vi "S4GUI_001.vi"() -> ()   [LabVIEW 2018] (continued)
  T9 = cluster{"Trigger Mode Status":string, "String output":string, "Instrument Status":cluster{"WPROT pos":dbl, "WPSEL pos":dbl, "GMIR pos":dbl, "GFOC pos":dbl, "CALW pos":dbl, "ASEL pos":dbl, "connection":bool, "mode":bool, "String Status":string}, "Sync Box State":i32, "Trigger General Status":string, "Instrument States":cluster{"WPSEL State":i32, "WPROT State":i32, "CALW State":i32, "ASEL State":i32, "GMIR State":i32, "GFOC State":i32}, "Instrument Pos Names":cluster{"WPROT posname":string, "WPSEL posname":string, "CALW posname":string, "ASEL posname":string}, "ChannelA_Status":cluster{"Current exp":dbl, "Frames done":u32, "LastFileImage":string, "CamStatus":string, "Run state":u32, "connection":bool, "Cooler ON/OFF":i16, "Currently temperature":i16, "Temperature Status":string, "target  temp":i16, "conf runing":bool, "FT":bool}, "WPROT seq":u16, "ChannelB_Status":cluster{"Current exp":dbl, "Frames done":u32, "LastFileImage":string, "CamStatus":string, "Run state":u32, "connection":bool, "Cooler ON/OFF":i16, "Currently temperature":i16, "Temperature Status":string, "target  temp":i16, "conf runing":bool, "FT":bool}, "ChannelC_Status":cluster{"Current exp":dbl, "Frames done":u32, "LastFileImage":string, "CamStatus":string, "Run state":u32, "connection":bool, "Cooler ON/OFF":i16, "Currently temperature":i16, "Temperature Status":string, "target  temp":i16, "conf runing":bool, "FT":bool}, "ChannelD_Status":cluster{"Current exp":dbl, "Frames done":u32, "LastFileImage":string, "CamStatus":string, "Run state":u32, "connection":bool, "Cooler ON/OFF":i16, "Currently temperature":i16, "Temperature Status":string, "target  temp":i16, "conf runing":bool, "FT":bool}, "ChannelA_CCD":cluster{"ACQUISITION_MODE":u8, "TRIGGER_MODE":u8, "READ_MODE":u8, "PREAMP":u8, "READOUT_RATE":u8, "VERTICAL_SHIFT_SPEED":u8, "EM_MODE":u8, "EM_GAIN":u16, "SHUTTER_MODE":u8, "SHUTTER_TTL":u8, "SHUTTER_OPENNING_TIME":u16, "SHUTTER_CLOSING_TIME":u16, "VBIN":u16, "HBIN":u16, "INITIAL_LINE":u16, "INITIAL_COLUMN":u16, "FINAL_LINE":u16, "FINAL_COLUMN":u16, "FRAME_TRANSFER":bool, "VERTICAL_CLOCK_VOLTAGE":u8, "AD_CHANNEL":u32}, "ChannelB_CCD ":cluster{"ACQUISITION_MODE":u8, "TRIGGER_MODE":u8, "READ_MODE":u8, "PREAMP":u8, "READOUT_RATE":u8, "VERTICAL_SHIFT_SPEED":u8, "EM_MODE":u8, "EM_GAIN":u16, "SHUTTER_MODE":u8, "SHUTTER_TTL":u8, "SHUTTER_OPENNING_TIME":u16, "SHUTTER_CLOSING_TIME":u16, "VBIN":u16, "HBIN":u16, "INITIAL_LINE":u16, "INITIAL_COLUMN":u16, "FINAL_LINE":u16, "FINAL_COLUMN":u16, "FRAME_TRANSFER":bool, "VERTICAL_CLOCK_VOLTAGE":u8, "AD_CHANNEL":u32}, "ChannelC_CCD":cluster{"ACQUISITION_MODE":u8, "TRIGGER_MODE":u8, "READ_MODE":u8, "PREAMP":u8, "READOUT_RATE":u8, "VERTICAL_SHIFT_SPEED":u8, "EM_MODE":u8, "EM_GAIN":u16, "SHUTTER_MODE":u8, "SHUTTER_TTL":u8, "SHUTTER_OPENNING_TIME":u16, "SHUTTER_CLOSING_TIME":u16, "VBIN":u16, "HBIN":u16, "INITIAL_LINE":u16, "INITIAL_COLUMN":u16, "FINAL_LINE":u16, "FINAL_COLUMN":u16, "FRAME_TRANSFER":bool, "VERTICAL_CLOCK_VOLTAGE":u8, "AD_CHANNEL":u32}, "ChannelD_CCD":cluster{"ACQUISITION_MODE":u8, "TRIGGER_MODE":u8, "READ_MODE":u8, "PREAMP":u8, "READOUT_RATE":u8, "VERTICAL_SHIFT_SPEED":u8, "EM_MODE":u8, "EM_GAIN":u16, "SHUTTER_MODE":u8, "SHUTTER_TTL":u8, "SHUTTER_OPENNING_TIME":u16, "SHUTTER_CLOSING_TIME":u16, "VBIN":u16, "HBIN":u16, "INITIAL_LINE":u16, "INITIAL_COLUMN":u16, "FINAL_LINE":u16, "FINAL_COLUMN":u16, "FRAME_TRANSFER":bool, "VERTICAL_CLOCK_VOLTAGE":u8, "AD_CHANNEL":u32}, "CHA_Checked Params":cluster{"ACQUISITION_MODE":bool, "TRIGGER_MODE":bool, "READ_MODE":bool, "PREAMP":bool, "READOUT_RATE":bool, "VERTICAL_SHIFT_SPEED":bool, "EM_MODE":bool, "EM_GAIN":bool, "SHUTTER_MODE":bool, "SHUTTER_TTL":bool, "SHUTTER_OPENING_TIME":bool, "SHUTTER_CLOSING_TIME":bool, "VBIN":bool, "HBIN":bool, "INITIAL_LINE":bool, "INITIAL_COLUMN":bool, "FINAL_LINE":bool, "FINAL_COLUMN":bool, "FRAME_TRANSFER":bool, "VERTICAL_CLOCK_VOLTAGE":bool, "AD_CHANNEL":bool}, "CHB_Checked Params":cluster{"ACQUISITION_MODE":bool, "TRIGGER_MODE":bool, "READ_MODE":bool, "PREAMP":bool, "READOUT_RATE":bool, "VERTICAL_SHIFT_SPEED":bool, "EM_MODE":bool, "EM_GAIN":bool, "SHUTTER_MODE":bool, "SHUTTER_TTL":bool, "SHUTTER_OPENING_TIME":bool, "SHUTTER_CLOSING_TIME":bool, "VBIN":bool, "HBIN":bool, "INITIAL_LINE":bool, "INITIAL_COLUMN":bool, "FINAL_LINE":bool, "FINAL_COLUMN":bool, "FRAME_TRANSFER":bool, "VERTICAL_CLOCK_VOLTAGE":bool, "AD_CHANNEL":bool}, "CHC_Checked Params":cluster{"ACQUISITION_MODE":bool, "TRIGGER_MODE":bool, "READ_MODE":bool, "PREAMP":bool, "READOUT_RATE":bool, "VERTICAL_SHIFT_SPEED":bool, "EM_MODE":bool, "EM_GAIN":bool, "SHUTTER_MODE":bool, "SHUTTER_TTL":bool, "SHUTTER_OPENING_TIME":bool, "SHUTTER_CLOSING_TIME":bool, "VBIN":bool, "HBIN":bool, "INITIAL_LINE":bool, "INITIAL_COLUMN":bool, "FINAL_LINE":bool, "FINAL_COLUMN":bool, "FRAME_TRANSFER":bool, "VERTICAL_CLOCK_VOLTAGE":bool, "AD_CHANNEL":bool}, "CHD_Checked Params":cluster{"ACQUISITION_MODE":bool, "TRIGGER_MODE":bool, "READ_MODE":bool, "PREAMP":bool, "READOUT_RATE":bool, "VERTICAL_SHIFT_SPEED":bool, "EM_MODE":bool, "EM_GAIN":bool, "SHUTTER_MODE":bool, "SHUTTER_TTL":bool, "SHUTTER_OPENING_TIME":bool, "SHUTTER_CLOSING_TIME":bool, "VBIN":bool, "HBIN":bool, "INITIAL_LINE":bool, "INITIAL_COLUMN":bool, "FINAL_LINE":bool, "FINAL_COLUMN":bool, "FRAME_TRANSFER":bool, "VERTICAL_CLOCK_VOLTAGE":bool, "AD_CHANNEL":bool}, "Trigger_connection":bool, "TCSPD_connection":bool, "TCS extended":string, "TCS id":u32}
  T10 = cluster{"Cluster Mode Sync":cluster{"#Index Cycles":enum8{"Enabled", "Disabled", "Disabled and Grayed Out"}, "#Cycles":enum8{"Enabled", "Disabled", "Disabled and Grayed Out"}, "SSM":enum8{"Enabled", "Disabled", "Disabled and Grayed Out"}, "Set SM":enum8{"Enabled", "Disabled", "Disabled and Grayed Out"}, "Star SM":enum8{"Enabled", "Disabled", "Disabled and Grayed Out"}, "Pause SM":enum8{"Enabled", "Disabled", "Disabled and Grayed Out"}, "Stop SM":enum8{"Enabled", "Disabled", "Disabled and Grayed Out"}, "Abort SM":enum8{"Enabled", "Disabled", "Disabled and Grayed Out"}, "Start SM Text":string}, "Cluster Polarimetry":cluster{"Lambda Selector":enum8{"Enabled", "Disabled", "Disabled and Grayed Out"}, "Calibrator Selector":enum8{"Enabled", "Disabled", "Disabled and Grayed Out"}, "Set Waveplate":enum8{"Enabled", "Disabled", "Disabled and Grayed Out"}, "Select Positions":enum8{"Enabled", "Disabled", "Disabled and Grayed Out"}, "P0":enum8{"Enabled", "Disabled", "Disabled and Grayed Out"}, "P1":enum8{"Enabled", "Disabled", "Disabled and Grayed Out"}, "P2":enum8{"Enabled", "Disabled", "Disabled and Grayed Out"}, "P3":enum8{"Enabled", "Disabled", "Disabled and Grayed Out"}, "P4":enum8{"Enabled", "Disabled", "Disabled and Grayed Out"}, "P5":enum8{"Enabled", "Disabled", "Disabled and Grayed Out"}, "P6":enum8{"Enabled", "Disabled", "Disabled and Grayed Out"}, "P7":enum8{"Enabled", "Disabled", "Disabled and Grayed Out"}, "P8":enum8{"Enabled", "Disabled", "Disabled and Grayed Out"}, "P9":enum8{"Enabled", "Disabled", "Disabled and Grayed Out"}, "P10":enum8{"Enabled", "Disabled", "Disabled and Grayed Out"}, "P11":enum8{"Enabled", "Disabled", "Disabled and Grayed Out"}, "P12":enum8{"Enabled", "Disabled", "Disabled and Grayed Out"}, "P13":enum8{"Enabled", "Disabled", "Disabled and Grayed Out"}, "P14":enum8{"Enabled", "Disabled", "Disabled and Grayed Out"}, "P15":enum8{"Enabled", "Disabled", "Disabled and Grayed Out"}}, "Cluster Mode CH1":cluster{"#cycles ch1":enum8{"Enabled", "Disabled", "Disabled and Grayed Out"}, "Start ch1":enum8{"Enabled", "Disabled", "Disabled and Grayed Out"}, "Pause ch1":enum8{"Enabled", "Disabled", "Disabled and Grayed Out"}, "Stop ch1":enum8{"Enabled", "Disabled", "Disabled and Grayed Out"}, "Abort ch1":enum8{"Enabled", "Disabled", "Disabled and Grayed Out"}, "Exptime ch1":enum8{"Enabled", "Disabled", "Disabled and Grayed Out"}, "Exp ch1":enum8{"Enabled", "Disabled", "Disabled and Grayed Out"}, "Start ch1 Text":string, "Set Cooler":enum8{"Enabled", "Disabled", "Disabled and Grayed Out"}, "Set Temp":enum8{"Enabled", "Disabled", "Disabled and Grayed Out"}}, "Cluster Mode CH2":cluster{"#cycles ch2":enum8{"Enabled", "Disabled", "Disabled and Grayed Out"}, "Start ch2":enum8{"Enabled", "Disabled", "Disabled and Grayed Out"}, "Pause ch2":enum8{"Enabled", "Disabled", "Disabled and Grayed Out"}, "Stop ch2":enum8{"Enabled", "Disabled", "Disabled and Grayed Out"}, "Abort ch2":enum8{"Enabled", "Disabled", "Disabled and Grayed Out"}, "Exptime ch2":enum8{"Enabled", "Disabled", "Disabled and Grayed Out"}, "Exp ch2":enum8{"Enabled", "Disabled", "Disabled and Grayed Out"}, "Start ch2 Text":string, "Set Cooler":enum8{"Enabled", "Disabled", "Disabled and Grayed Out"}, "Set Temp":enum8{"Enabled", "Disabled", "Disabled and Grayed Out"}}, "Cluster Mode CH3":cluster{"#cycles ch3":enum8{"Enabled", "Disabled", "Disabled and Grayed Out"}, "Start ch3":enum8{"Enabled", "Disabled", "Disabled and Grayed Out"}, "Pause ch3":enum8{"Enabled", "Disabled", "Disabled and Grayed Out"}, "Stop ch3":enum8{"Enabled", "Disabled", "Disabled and Grayed Out"}, "Abort ch3":enum8{"Enabled", "Disabled", "Disabled and Grayed Out"}, "Exptime ch3":enum8{"Enabled", "Disabled", "Disabled and Grayed Out"}, "Exp ch3":enum8{"Enabled", "Disabled", "Disabled and Grayed Out"}, "Start ch3 Text":string, "Set Cooler":enum8{"Enabled", "Disabled", "Disabled and Grayed Out"}, "Set Temp":enum8{"Enabled", "Disabled", "Disabled and Grayed Out"}}, "Cluster Mode CH4":cluster{"#cycles ch4":enum8{"Enabled", "Disabled", "Disabled and Grayed Out"}, "Start ch4":enum8{"Enabled", "Disabled", "Disabled and Grayed Out"}, "Pause ch4":enum8{"Enabled", "Disabled", "Disabled and Grayed Out"}, "Stop ch4":enum8{"Enabled", "Disabled", "Disabled and Grayed Out"}, "Abort ch4":enum8{"Enabled", "Disabled", "Disabled and Grayed Out"}, "Exptime ch4":enum8{"Enabled", "Disabled", "Disabled and Grayed Out"}, "Exp ch4":enum8{"Enabled", "Disabled", "Disabled and Grayed Out"}, "Start ch4 Text":string, "Set Cooler":enum8{"Enabled", "Disabled", "Disabled and Grayed Out"}, "Set Temp":enum8{"Enabled", "Disabled", "Disabled and Grayed Out"}}, "Cluster ExpMode":cluster{"tab4":enum8{"Enabled", "Disabled", "Disabled and Grayed Out"}}}
  T11 = cluster{"WPROT pos":dbl, "WPSEL pos":dbl, "GMIR pos":dbl, "GFOC pos":dbl, "CALW pos":dbl, "ASEL pos":dbl, "connection":bool, "mode":bool, "String Status":string}
  T12 = cluster{"WPSEL State":i32, "WPROT State":i32, "CALW State":i32, "ASEL State":i32, "GMIR State":i32, "GFOC State":i32}
  T13 = cluster{"WPROT posname":string, "WPSEL posname":string, "CALW posname":string, "ASEL posname":string}
  T14 = cluster{"Current exp":dbl, "Frames done":u32, "LastFileImage":string, "CamStatus":string, "Run state":u32, "connection":bool, "Cooler ON/OFF":i16, "Currently temperature":i16, "Temperature Status":string, "target  temp":i16, "conf runing":bool, "FT":bool}
  T15 = cluster{"Lambda Selector":enum8{"Enabled", "Disabled", "Disabled and Grayed Out"}, "Calibrator Selector":enum8{"Enabled", "Disabled", "Disabled and Grayed Out"}, "Set Waveplate":enum8{"Enabled", "Disabled", "Disabled and Grayed Out"}, "Select Positions":enum8{"Enabled", "Disabled", "Disabled and Grayed Out"}, "P0":enum8{"Enabled", "Disabled", "Disabled and Grayed Out"}, "P1":enum8{"Enabled", "Disabled", "Disabled and Grayed Out"}, "P2":enum8{"Enabled", "Disabled", "Disabled and Grayed Out"}, "P3":enum8{"Enabled", "Disabled", "Disabled and Grayed Out"}, "P4":enum8{"Enabled", "Disabled", "Disabled and Grayed Out"}, "P5":enum8{"Enabled", "Disabled", "Disabled and Grayed Out"}, "P6":enum8{"Enabled", "Disabled", "Disabled and Grayed Out"}, "P7":enum8{"Enabled", "Disabled", "Disabled and Grayed Out"}, "P8":enum8{"Enabled", "Disabled", "Disabled and Grayed Out"}, "P9":enum8{"Enabled", "Disabled", "Disabled and Grayed Out"}, "P10":enum8{"Enabled", "Disabled", "Disabled and Grayed Out"}, "P11":enum8{"Enabled", "Disabled", "Disabled and Grayed Out"}, "P12":enum8{"Enabled", "Disabled", "Disabled and Grayed Out"}, "P13":enum8{"Enabled", "Disabled", "Disabled and Grayed Out"}, "P14":enum8{"Enabled", "Disabled", "Disabled and Grayed Out"}, "P15":enum8{"Enabled", "Disabled", "Disabled and Grayed Out"}}
  T16 = cluster{"#Index Cycles":enum8{"Enabled", "Disabled", "Disabled and Grayed Out"}, "#Cycles":enum8{"Enabled", "Disabled", "Disabled and Grayed Out"}, "SSM":enum8{"Enabled", "Disabled", "Disabled and Grayed Out"}, "Set SM":enum8{"Enabled", "Disabled", "Disabled and Grayed Out"}, "Star SM":enum8{"Enabled", "Disabled", "Disabled and Grayed Out"}, "Pause SM":enum8{"Enabled", "Disabled", "Disabled and Grayed Out"}, "Stop SM":enum8{"Enabled", "Disabled", "Disabled and Grayed Out"}, "Abort SM":enum8{"Enabled", "Disabled", "Disabled and Grayed Out"}, "Start SM Text":string}
  T17 = cluster{"#cycles ch1":enum8{"Enabled", "Disabled", "Disabled and Grayed Out"}, "Start ch1":enum8{"Enabled", "Disabled", "Disabled and Grayed Out"}, "Pause ch1":enum8{"Enabled", "Disabled", "Disabled and Grayed Out"}, "Stop ch1":enum8{"Enabled", "Disabled", "Disabled and Grayed Out"}, "Abort ch1":enum8{"Enabled", "Disabled", "Disabled and Grayed Out"}, "Exptime ch1":enum8{"Enabled", "Disabled", "Disabled and Grayed Out"}, "Exp ch1":enum8{"Enabled", "Disabled", "Disabled and Grayed Out"}, "Start ch1 Text":string, "Set Cooler":enum8{"Enabled", "Disabled", "Disabled and Grayed Out"}, "Set Temp":enum8{"Enabled", "Disabled", "Disabled and Grayed Out"}}
  T18 = cluster{"#cycles ch2":enum8{"Enabled", "Disabled", "Disabled and Grayed Out"}, "Start ch2":enum8{"Enabled", "Disabled", "Disabled and Grayed Out"}, "Pause ch2":enum8{"Enabled", "Disabled", "Disabled and Grayed Out"}, "Stop ch2":enum8{"Enabled", "Disabled", "Disabled and Grayed Out"}, "Abort ch2":enum8{"Enabled", "Disabled", "Disabled and Grayed Out"}, "Exptime ch2":enum8{"Enabled", "Disabled", "Disabled and Grayed Out"}, "Exp ch2":enum8{"Enabled", "Disabled", "Disabled and Grayed Out"}, "Start ch2 Text":string, "Set Cooler":enum8{"Enabled", "Disabled", "Disabled and Grayed Out"}, "Set Temp":enum8{"Enabled", "Disabled", "Disabled and Grayed Out"}}
  T19 = cluster{"#cycles ch3":enum8{"Enabled", "Disabled", "Disabled and Grayed Out"}, "Start ch3":enum8{"Enabled", "Disabled", "Disabled and Grayed Out"}, "Pause ch3":enum8{"Enabled", "Disabled", "Disabled and Grayed Out"}, "Stop ch3":enum8{"Enabled", "Disabled", "Disabled and Grayed Out"}, "Abort ch3":enum8{"Enabled", "Disabled", "Disabled and Grayed Out"}, "Exptime ch3":enum8{"Enabled", "Disabled", "Disabled and Grayed Out"}, "Exp ch3":enum8{"Enabled", "Disabled", "Disabled and Grayed Out"}, "Start ch3 Text":string, "Set Cooler":enum8{"Enabled", "Disabled", "Disabled and Grayed Out"}, "Set Temp":enum8{"Enabled", "Disabled", "Disabled and Grayed Out"}}
  T20 = cluster{"#cycles ch4":enum8{"Enabled", "Disabled", "Disabled and Grayed Out"}, "Start ch4":enum8{"Enabled", "Disabled", "Disabled and Grayed Out"}, "Pause ch4":enum8{"Enabled", "Disabled", "Disabled and Grayed Out"}, "Stop ch4":enum8{"Enabled", "Disabled", "Disabled and Grayed Out"}, "Abort ch4":enum8{"Enabled", "Disabled", "Disabled and Grayed Out"}, "Exptime ch4":enum8{"Enabled", "Disabled", "Disabled and Grayed Out"}, "Exp ch4":enum8{"Enabled", "Disabled", "Disabled and Grayed Out"}, "Start ch4 Text":string, "Set Cooler":enum8{"Enabled", "Disabled", "Disabled and Grayed Out"}, "Set Temp":enum8{"Enabled", "Disabled", "Disabled and Grayed Out"}}
  T21 = cluster{"ACQUISITION_MODE":u8, "TRIGGER_MODE":u8, "READ_MODE":u8, "PREAMP":u8, "READOUT_RATE":u8, "VERTICAL_SHIFT_SPEED":u8, "EM_MODE":u8, "EM_GAIN":u16, "SHUTTER_MODE":u8, "SHUTTER_TTL":u8, "SHUTTER_OPENNING_TIME":u16, "SHUTTER_CLOSING_TIME":u16, "VBIN":u16, "HBIN":u16, "INITIAL_LINE":u16, "INITIAL_COLUMN":u16, "FINAL_LINE":u16, "FINAL_COLUMN":u16, "FRAME_TRANSFER":bool, "VERTICAL_CLOCK_VOLTAGE":u8, "AD_CHANNEL":u32}
  T22 = cluster{"ACQUISITION_MODE":bool, "TRIGGER_MODE":bool, "READ_MODE":bool, "PREAMP":bool, "READOUT_RATE":bool, "VERTICAL_SHIFT_SPEED":bool, "EM_MODE":bool, "EM_GAIN":bool, "SHUTTER_MODE":bool, "SHUTTER_TTL":bool, "SHUTTER_OPENING_TIME":bool, "SHUTTER_CLOSING_TIME":bool, "VBIN":bool, "HBIN":bool, "INITIAL_LINE":bool, "INITIAL_COLUMN":bool, "FINAL_LINE":bool, "FINAL_COLUMN":bool, "FRAME_TRANSFER":bool, "VERTICAL_CLOCK_VOLTAGE":bool, "AD_CHANNEL":bool}
  T23 = cluster{"Image \nInitial Line":u16, "Image\nInitial Column":u16, "Image\nFinal Line":u16, "Image\nFInal Column":u16, "Vertical\nBinning":u16, "Horizontal\nBinning":u16, "Pre-amplification\nGain":u8, "CCD\nEM Gain":u16, "Readout\nRate":u8, "Shutter\nOpenning Time":i32, "Shutter\nClosing Time":i32, "Vertical\nShift Speed":u8, "Read\nMode":u8, "Vertical\nClock Voltage":u8, "A/D \nChannel":u32, "Shutter\nMode":u16, "Shutter\nTTL":u16, "Trigger\nMode":u16, "Frame\nTransfer":bool, "Acquisition\nMode":u8, "CCD \nEM Mode":u8}
  T24 = cluster{"ACQUISITION_MODE":u8, "TRIGGER_MODE":u8, "READ_MODE":u8, "PREAMP":u8, "READOUT_RATE":u8, "VERTICAL_SHIFT_SPEED":u8, "EM_MODE":u8, "EM_GAIN":u16, "SHUTTER_MODE":u8, "SHUTTER_TTL":u8, "SHUTTER_OPENING_TIME":u16, "SHUTTER_CLOSING_TIME":u16, "VBIN":u16, "HBIN":u16, "INITIAL_LINE":u16, "INITIAL_COLUMN":u16, "FINAL_LINE":u16, "FINAL_COLUMN":u16, "FRAME_TRANSFER":bool, "VERTICAL_CLOCK_VOLTAGE":u8, "AD_CHANNEL":u32}
  T25 = cluster{"Image Initial Line":dbl, "Image Initial Column":dbl, "Image Final Line":dbl, "Image FInal Column":dbl, "Vertical Binning":dbl, "Horizontal Binning":dbl, "Pre-amplification Gain":u8, "CCD EM Gain":u8, "Readout Rate":u8, "Shutter Openning Time":i32, "Shutter Closing Time":i32, "Vertical Shift Speed":u8, "Read Mode":u8, "Vertical Clock Voltage":u8, "A/D  Channel":u32, "Image Initial Line 2":dbl, "Image Initial Column 2":dbl, "Image Final Line 2":dbl, "Image FInal Column 2":dbl, "Vertical Binning 2":dbl, "Horizontal Binning 2":dbl, "Pre-amplification Gain 2":u8, "CCD EM Gain 2":u16, "Readout Rate 2":u8, "Shutter Openning Time 2":i32, "Shutter Closing Time 2":i32, "Vertical Shift Speed 2":u8, "Read Mode 2":u8, "Vertical Clock Voltage 2":u8, "A/D Channel 2":u32, "Image Initial Line 3":dbl, "Image Initial Column 3":dbl, "Image Final Line 3":dbl, "Image FInal Column 3":dbl, "Vertical Binning 3":dbl, "Horizontal Binning 3":dbl, "Pre-amplification Gain 3":u8, "CCD EM Gain 3":u16, "Readout Rate 3":u8, "Shutter Openning Time 3":i32, "Shutter Closing Time 3":i32, "Vertical Shift Speed 3":u8, "Read Mode 3":u8, "Vertical Clock Voltage 3":u8, "A/D Channel 3":u32, "Image Initial Line 4":dbl, "Image Initial Column 4":dbl, "Image Final Line 4":dbl, "Image FInal Column 4":dbl, "Vertical Binning 4":dbl, "Horizontal Binning 4":dbl, "Pre-amplification Gain 4":u8, "CCD EM Gain 4":u16, "Readout Rate 4":u8, "Shutter Openning Time 4":i32, "Shutter Closing Time 4":i32, "Vertical Shift Speed 4":u8, "Read Mode 4":u8, "Vertical Clock Voltage 4":u8, "A/D Channel 4":u32, "CCD EM Mode 2":u8, "CCD EM Mode 3":u8, "CCD EM Mode 4":u8, "CCD EM Mode":u16, "Shutter Mode":u16, "Shutter Mode 2":u16, "Shutter Mode 4":u16, "Shutter Mode 3":u16, "Shutter TTL":u16, "Shutter TTL 2":u16, "Shutter TTL 3":u16, "Shutter TTL 4":u16, "Frame Transfer":bool, "Frame Transfer 2":bool, "Frame Transfer 3":bool, "Frame Transfer 4":bool, "Trigger Mode":u16, "Trigger Mode 2":u16, "Trigger Mode 3":u16, "Trigger Mode 4":u16, "Acquisition Mode":u8, "Acquisition Mode 2":u8, "Acquisition Mode 3":u8, "Acquisition Mode 4":u8}
diagram:
  w6 = T7."Disabled" ("Disabled")
  (unwired) -580 ("Position:Top")
  (unwired) -400 ("Position:Top")
  w11 = "" ("Temp Status 1")
  w12 = i16 0 ("Curr Temp 1")
  w13 = FALSE ("Cooler status 1")
  w14 = u16 1 items=["Asynchronous", "Synchronous by Cycle"] ("SSM")
  (unwired) -400 ("Position:Top")
  (unwired) -580 ("Position:Top")
  w25 = u16 4 items=["All 16 positions", "First 8 positions", "First 4 positions", "1-4 & 9-12", "Clear", "Customized"] ("Select Positions")
  w5 = FALSE
  n1 = local write "Select Positions"(w25) -> ()
  n2 = property on="Tab Acq Type" class="TabCtl (strict)"("DisabledEnum"=T7."Disabled and Grayed Out" ("Disabled")) -> ()  [unwired: 2 in, 2 out]
  n3 = property on="Tab ObsEng" class="TabCtl (strict)"("Visible"=TRUE) -> ()  [unwired: 2 in, 2 out]
  n4 = flat-sequence {
    tunnel: errorcluster {"status"=FALSE, "code"=0, "source"=""} ("error in (no error)") -> [w30]
    tunnel: [w30] -> w8
    frame #0 {
      w31 = u32 240 ("Tab Control Pane Dimension:Width")
      w32 = u32 300 ("Tab Control Pane Dimension:Height")
      n5 = property on="Tab CH2" class="TabCtl (strict)"("PaneHeight"=w32, "PaneWidth"=w31) -> ()  [unwired: 2 in, 2 out]
      n6 = property on="Tab CH1" class="TabCtl (strict)"("PaneHeight"=w32, "PaneWidth"=w31) -> ()  [unwired: 2 in, 2 out]
      n7 = property on="Tab CH3" class="TabCtl (strict)"("PaneHeight"=w32, "PaneWidth"=w31) -> ()  [unwired: 2 in, 2 out]
      n8 = property on="Tab CH4" class="TabCtl (strict)"("PaneHeight"=w32, "PaneWidth"=w31) -> ()  [unwired: 2 in, 2 out]
      n9 = local write "loop max(ms)"(u32 0 ("loop max(ms)")) -> ()
    }
  }
  n10 = property on="SSM" class="Ring (strict)"("Value"=w14) -> ()  [unwired: 2 in, 2 out]
  n11 = disable-structure shown="Enabled" {
    disable-tunnel: "S4ACS_GUI.lvclass" -> [w41 w42]
    disable-tunnel: [w38 w42] -> w17
    disable-tunnel: w8 -> [w40 w43]
    disable-tunnel: [w39 w43] -> w16
    frame Enabled {
      # "Carrega o ultimo filtro escolhido para os 4 canais."
      n12 = local read "Filter1"() -> (w37:u8)
      n13 = local read "Filter2"() -> (w36:u8)
      n14 = local read "Filter3"() -> (w35:u8)
      n15 = local read "Filter4"() -> (w34:u8)
      n16 = call-dynamic "LoadFilters.vi"("Filter 4"=w34, "Filter 3"=w35, "error in (no error)"=w40, "Filter 2"=w36, "Filter 1"=w37, "S4GUI in"=w41) -> ("error out"=w39:errorcluster, "S4GUI out"=w38:refnum<class "S4GUI.lvclass">)  [unwired: 4 in]
    }
    frame Disabled {
    }
  }
  n17 = flat-sequence "Indicadores dos canais da parte inferior da tela principal" {
    frame #0 {
      w44 = ""
      "B1" <- w44
      "PA1" <- w44
      "RO1" <- w44
      "G1" <- w44
      "SI2" <- w44
      "PA2" <- w44
      "G2" <- w44
      "B2" <- w44
      "RO2" <- w44
      "EA2" <- w44
      "SI3" <- w44
      "EA3" <- w44
      "PA3" <- w44
      "B3" <- w44
      "G3" <- w44
      "RO3" <- w44
      "SI4" <- w44
      "EA4" <- w44
      "PA4" <- w44
      "B4" <- w44
      "G4" <- w44
      "RO4" <- w44
      "SI1" <- w44
      "EA1" <- w44
    }
  }
  n18 = local write "Cooler status 4"(w13) -> ()
  n19 = local write "Curr Temp 4"(w12) -> ()
  n20 = local write "Panel Temp 4"(w12) -> ()
  n21 = local write "Temp Status 4"(w11) -> ()
  n22 = local write "Panel cooler 1"(w13) -> ()
  n23 = local write "Panel cooler 4"(w13) -> ()
  n24 = local write "Cooler status 1"(w13) -> ()
  n25 = local write "Curr Temp 1"(w12) -> ()
  n26 = local write "Panel Temp"(w12) -> ()
  n27 = local write "Temp Status 1"(w11) -> ()
  n28 = local write "Panel cooler 2"(w13) -> ()
  n29 = local write "Curr Temp 2"(w12) -> ()
  n30 = local write "Panel Temp 2"(w12) -> ()
  n31 = local write "Temp Status 2"(w11) -> ()
  n32 = local write "Panel cooler 3"(w13) -> ()
  n33 = local write "Cooler status 3"(w13) -> ()
  n34 = local write "Curr Temp 3"(w12) -> ()
  n35 = local write "Panel Temp 3"(w12) -> ()
  n36 = local write "Temp Status 3"(w11) -> ()
  n37 = control-ref of="Current Configuration"() -> (w23:refnum<vi>)
  n38 = local write "Cooler status 2"(w13) -> ()
  n39 = control-ref of="Parameters"() -> (w20:refnum<vi>)
  n40 = property on="Property Node" class="Clust (strict)"(reference=w20, "Top"=230 ("Position:Top")) -> (reference out=w24:refnum<vi>)  [unwired: 1 in, 1 out]
  n41 = property on="Property Node" class="Clust (strict)"(reference=w23, "Top"=230 ("Position:Top")) -> (reference out=w22:refnum<vi>)  [unwired: 1 in, 1 out]
  n42 = disable-structure shown="Enabled" {
    frame Enabled {
      n43 = property on="Observer" class="Str"("Value"="" ("Observer"), "Text.BGColor"=u32 16448250) -> ()  [unwired: 2 in, 2 out]
    }
    frame Disabled {
    }
  }
  n44 = property on="ExtSync" class="Bool (strict)"("Value"=FALSE ("ExtSync")) -> ()  [unwired: 2 in, 2 out]
  n45 = local write "GUIDER"(FALSE ("GUIDER")) -> ()
  n46 = local write "rotator"(0.0 ("rotator")) -> ()
  n47 = property on="Object_dflat" class="Str"("DisabledEnum"=w6) -> ()  [unwired: 2 in, 2 out]
  n48 = property on="Object_zero" class="Str"("DisabledEnum"=w6) -> ()  [unwired: 2 in, 2 out]
  n49 = property on="Object_sflat" class="Str"("DisabledEnum"=w6) -> ()  [unwired: 2 in, 2 out]
  n50 = Bundle("Parameters"=w24, "Current Configuration"=w22) -> (w21:T8)  [unwired: 1 in]
  n51 = call-dynamic "Initialize.vi"("error in (no error)"=w16, "S4ACS_GUI in"=w17) -> ("error out"=w28:errorcluster, "S4ACS_GUI out"=w29:refnum<class "S4GUI.lvclass">)  [unwired: 8 in]
  n52 = local write "P8"(w5) -> ()
  n53 = local write "P9"(w5) -> ()
  n54 = local write "P10"(w5) -> ()
  n55 = local write "P11"(w5) -> ()
  n56 = local write "P12"(w5) -> ()
  n57 = local write "P13"(w5) -> ()
  n58 = local write "P14"(w5) -> ()
  n59 = local write "P15"(w5) -> ()
  n60 = local write "P1"(w5) -> ()
  n61 = local write "P2"(w5) -> ()
  n62 = local write "P3"(w5) -> ()
  n63 = local write "P4"(w5) -> ()
  n64 = local write "P5"(w5) -> ()
  n65 = local write "P6"(w5) -> ()
  n66 = local write "P7"(w5) -> ()
  n67 = local write "P0"(TRUE ("P0")) -> ()
  n68 = while {
    shift-right: [w55] -> w27
    shift-left: w29 -> [w58]
    shift-right: [w67] -> _
    shift-left: w28 -> [w68]
    tunnel: w21 -> [w63]
    i -> [w48]
    stop <- w66 stop-if-true
    # "Sufixo do arquivo SEMPRE\nem minúsculas."
    n69 = case shown="\"OBJECT\", Default" "Tab Acq Type" {
      tunnel: ["object suffix" "dflat suffix" "sflat suffix" "dark suffix" "zero suffix" "focus suffix"] -> w50
      tunnel: ["OBJECT Comments" "DFLAT Comments" "SFLAT Comments" "DARK Comments" "ZERO Comments" "FOCUS Comments"] -> w64
      tunnel: ["OBJECT" "FLAT" "FLAT" "DARK" "ZERO" "FOCUS"] -> w61
      tunnel: ["Object_obj" "DOMEFLAT" "SKYFLAT" "Object_dark" "ZERO" "Object_focus"] -> w60
      frame "OBJECT", Default {
      }
      frame "DFLAT" {
      }
      frame "SFLAT" {
      }
      frame "DARK" {
      }
      frame "ZERO" {
      }
      frame "FOCUS" {
      }
    }
    n70 = flat-sequence {
      tunnel: w58 -> [w81]
      tunnel: [w81] -> w57
      tunnel: [w80] -> w54
      frame #0 {
        n71 = case shown="True" "reset max" {
          frame False {
          }
          frame True {
            n72 = local write "loop max(ms)"(u32 0 ("loop max(ms)")) -> ()
          }
        }
        n73 = Tick Count (ms)() -> (millisecond timer value=w80:u32)
      }
    }
    n74 = To Lower Case(string=w50) -> (all lower case string=w49:string)
    n75 = event shown="[35] \"Start ch1\": Value Change" {
      selector: _ -> [_ _ _ _ _ _ _ _ _ _ _ _ _ _ _ _ _ _ _ _ _ _ _ _ _ _ _ _ _ _ _ _ _ _ _ _ _ _ _ _ _ _ _ _ _ _ _ _ _ _ _ _ _ _ _ _ _ _ _ _ _ _ _ _ _ _ _ _ _ _ _ _ _ _ _ _ _ _ _ _ _ _ _ _ _ _ _ _ _ _ _ _ _ _ _ _ _ _ _ _ _ _ _ _ _ _ _ _ _ _]
      dyn-events: _ -> [_ _ _ _ _ _ _ _ _ _ _ _ _ _ _ _ _ _ _ _ _ _ _ _ _ _ _ _ _ _ _ _ _ _ _ _ _ _ _ _ _ _ _ _ _ _ _ _ _ _ _ _ _ _ _ _ _ _ _ _ _ _ _ _ _ _ _ _ _ _ _ _ _ _ _ _ _ _ _ _ _ _ _ _ _ _ _ _ _ _ _ _ _ _ _ _ _ _ _ _ _ _ _ _ _ _ _ _ _ _]
      timeout: 20 -> [_ _ _ _ _ _ _ _ _ _ _ _ _ _ _ _ _ _ _ _ _ _ _ _ _ _ _ _ _ _ _ _ _ _ _ _ _ _ _ _ _ _ _ _ _ _ _ _ _ _ _ _ _ _ _ _ _ _ _ _ _ _ _ _ _ _ _ _ _ _ _ _ _ _ _ _ _ _ _ _ _ _ _ _ _ _ _ _ _ _ _ _ _ _ _ _ _ _ _ _ _ _ _ _ _ _ _ _ _ _]
      tunnel: w57 -> [w138 w1536 w1547 w1620 w1706 w1775 w1844 w1876 w1891 w2017 w2196 w2228 w2260 w2292 w2326 w2360 w2394 w2431 w2434 w2468 w2610 w2665 w3181 w3222 w3257 w3651 w3657 w3747 w4833 w5074 w5255 w5444 w5627 w5822 w5837 w6018 w6147 w6273 w6400 w6522 w6542 w6563 w6628 w6693 w6758 w6823 w6860 w6888 w6916 w6946 w7016 w7141 w7173 w7232 w7291 w7350 w7409 w7429 w7456 w7472 w7493 w7520 w7547 w7574 w7601 w7628 w7663 w7698 w7733 w7773 w7793 w7808 w7823 w7838 w7853 w7868 w7883 w7898 w7929 w7958 w7982 w8024 w8058 w8086 w8112 w8140 w8160 w8175 w8195 w8264 w8598 w8633 w8653 w8673 w8688 w8708 w8728 w8748 w8763 w8783 w8803 w8823 w8838 w8858 w8878 w8898 w8913 w8933 w8953 w8973]
      tunnel: w68 -> [w137 w1535 w1546 w1619 w1705 w1774 w1843 w1875 w1882 w2008 w2195 w2227 w2259 w2291 w2325 w2359 w2393 w2430 w2442 w2469 w2609 w2664 w3172 w3220 w3256 w3650 w3656 w3746 w4832 w5073 w5254 w5443 w5620 w5820 w5836 w6016 w6146 w6271 w6399 w6523 w6543 w6562 w6627 w6692 w6757 w6821 w6858 w6886 w6914 w6945 w7015 w7140 w7172 w7231 w7290 w7349 w7408 w7428 w7455 w7471 w7492 w7519 w7546 w7573 w7600 w7627 w7662 w7697 w7732 w7772 w7792 w7807 w7822 w7837 w7852 w7867 w7882 w7897 w7928 w7957 w7981 w8023 w8057 w8085 w8111 w8139 w8159 w8174 w8194 w8265 w8597 w8632 w8652 w8672 w8687 w8707 w8727 w8747 w8762 w8782 w8802 w8822 w8837 w8857 w8877 w8897 w8912 w8932 w8952 w8972]
      tunnel: [w108 w1523 w1551 w1619 w1646 w1715 w1784 w1862 w1889 w2015 w2106 w2214 w2246 w2278 w2316 w2350 w2384 w2421 w2442 w2454 w2574 w2658 w3086 w3223 w3250 w3649 w3653 w3772 w4877 w5067 w5248 w5437 w5621 w5821 w5829 w6012 w6156 w6282 w6409 w6521 w6541 w6561 w6626 w6691 w6756 w6822 w6859 w6887 w6915 w6944 w7014 w7138 w7171 w7230 w7289 w7348 w7407 w7427 w7454 w7470 w7491 w7518 w7545 w7572 w7599 w7626 w7661 w7696 w7731 w7771 w7791 w7806 w7821 w7836 w7851 w7866 w7881 w7896 w7913 w7955 w7980 w8022 w8056 w8084 w8110 w8122 w8142 w8162 w8178 w8202 w8599 w8618 w8635 w8655 w8675 w8693 w8710 w8730 w8750 w8766 w8785 w8805 w8825 w8841 w8860 w8880 w8900 w8916 w8935 w8955] -> w67
      tunnel: [w134 _ _ _ _ _ _ _ _ _ _ _ _ _ _ _ _ _ _ _ _ _ _ _ _ _ _ _ _ _ _ _ _ _ _ _ _ _ _ _ _ _ _ _ _ _ _ _ _ _ _ _ _ _ _ _ _ _ _ _ _ _ _ _ _ _ _ _ _ _ _ _ _ _ _ _ _ _ _ _ _ _ _ _ _ _ _ _ _ _ _ _ _ _ _ _ _ _ _ _ _ _ _ _ _ _ _ _ _ _] -> w66
      tunnel: w49 -> [_ _ _ _ _ _ _ _ _ _ _ _ _ _ _ _ _ _ _ _ _ _ _ _ w3249 _ _ _ _ w5072 w5252 _ w5625 _ w5834 w6025 w6155 w6281 w6408 _ _ _ _ _ _ _ _ _ _ _ _ _ _ _ _ _ _ _ _ _ _ _ _ _ _ _ _ _ _ _ _ _ _ _ _ _ _ _ _ _ _ _ _ _ _ _ _ _ _ _ _ _ _ _ _ _ _ _ _ _ _ _ _ _ _ _ _ _ _ _]
      tunnel: w64 -> [_ _ _ _ _ _ _ _ _ _ _ _ _ _ _ _ _ _ _ _ _ _ _ _ w3248 _ _ _ _ w5071 _ w5441 w5624 _ w5833 w6024 w6154 w6280 w6407 _ _ _ _ _ _ _ _ _ _ _ _ _ _ _ _ _ _ _ _ _ _ _ _ _ _ _ _ _ _ _ _ _ _ _ _ _ _ _ _ _ _ _ _ _ _ _ _ _ _ _ _ _ _ _ _ _ _ _ _ _ _ _ _ _ _ _ _ _ _ _]
      tunnel: w63 -> [_ _ _ _ _ _ _ _ _ _ _ _ _ _ _ _ _ _ w2435 _ _ _ _ _ _ _ _ _ _ _ _ _ _ _ _ _ _ _ _ _ _ _ _ _ _ _ _ _ _ _ _ _ _ _ _ _ _ _ _ _ _ _ _ _ _ _ _ _ _ _ _ _ _ _ _ _ _ _ _ _ _ _ _ _ _ _ _ _ _ _ _ _ _ _ _ _ _ _ _ _ _ _ _ _ _ _ _ _ _ _]
      tunnel: [w109 w1524 w1552 w1620 w1647 w1716 w1785 w1853 w1890 w2016 w2108 w2205 w2237 w2269 w2293 w2327 w2361 w2398 w2434 w2453 w2575 w2671 w3087 w3224 w3247 w3648 w3652 w3771 w4876 w5068 w5249 w5438 w5622 w5822 w5830 w6013 w6153 w6279 w6406 w6520 w6540 w6560 w6625 w6690 w6755 w6820 w6857 w6885 w6913 w6942 w7012 w7139 w7170 w7229 w7288 w7347 w7406 w7426 w7446 w7469 w7490 w7517 w7544 w7571 w7598 w7625 w7660 w7695 w7730 w7764 w7787 w7802 w7817 w7832 w7847 w7862 w7877 w7892 w7912 w7930 w7967 w7991 w8039 w8070 w8098 w8121 w8141 w8161 w8176 w8203 w8600 w8614 w8634 w8654 w8674 w8691 w8709 w8729 w8749 w8764 w8784 w8804 w8824 w8839 w8859 w8879 w8899 w8914 w8934 w8954] -> w56
      tunnel: "Input Cluster" -> [_ _ _ _ _ _ _ _ _ _ _ _ _ _ _ _ _ w2397 w2433 _ _ _ _ _ _ _ _ _ _ _ _ _ _ _ _ _ _ _ _ _ _ _ _ _ _ _ _ _ _ _ _ _ _ _ _ _ _ _ _ _ _ _ _ _ _ _ _ _ _ _ _ _ _ _ _ _ _ _ _ _ _ _ _ _ _ _ _ _ _ _ _ _ _ _ _ _ _ _ _ _ _ _ _ _ _ _ _ _ _ _]
      tunnel: w61 -> [_ _ _ _ _ _ _ _ _ _ _ _ _ _ _ _ _ _ _ _ _ _ _ _ w3246 _ _ _ _ w5069 w5250 w5439 w5623 _ w5831 w6023 w6152 w6277 w6405 _ _ _ _ _ _ _ _ _ _ _ _ _ _ _ _ _ _ _ _ _ _ _ _ _ _ _ _ _ _ _ _ _ _ _ _ _ _ _ _ _ _ _ _ _ _ _ _ _ _ _ _ _ _ _ _ _ _ _ _ _ _ _ _ _ _ _ _ _ _ _]
      tunnel: w60 -> [_ _ _ _ _ _ _ _ _ _ _ _ _ _ _ _ _ _ _ _ _ _ _ _ w3245 _ _ _ _ _ w5253 w5442 w5626 _ w5835 w6022 w6151 w6278 w6404 _ _ _ _ _ _ _ _ _ _ _ _ _ _ _ _ _ _ _ _ _ _ _ _ _ _ _ _ _ _ _ _ _ _ _ _ _ _ _ _ _ _ _ _ _ _ _ _ _ _ _ _ _ _ _ _ _ _ _ _ _ _ _ _ _ _ _ _ _ _ _]
